vi "Set Server State Ref.vi"(10 "Server Internal State Ref":refnum<data-value>, 11 "Template Server in":refnum<class "HVC.lvclass">) -> (3 "Template Server out":refnum<class "HVC.lvclass">)   [LabVIEW 2019, in "HVC.lvlib" / "HVC.lvclass"]
uses:
  HVC.lvclass
  typeDefs/Server State Data.ctl
  HVC.lvclass/HVC.ctl
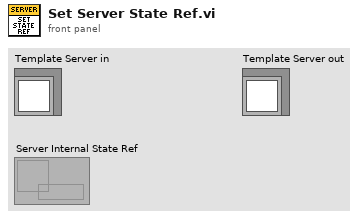
[diagram p1: front panel]
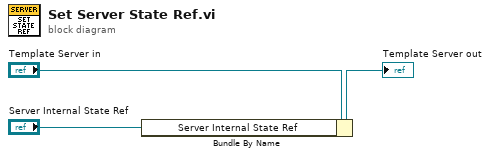
[diagram p0: block diagram]
diagram:
  n1 = Bundle By Name(cluster="Template Server in", "Server Internal State Ref"="Server Internal State Ref") -> (→"Template Server out":refnum<class "HVC.lvclass">)
